vi "Counter - Count Edges Test.vi"(10 "Sample Rate":dbl=100000.0, 11 "Samples per Loop":i32=100) -> (1 "counts/bin":u32[](array[numeric]), 2 "raw Data":u32[](array[numeric]))   [LabVIEW 2022 SP3]
doc: "This example demonstrates how to continuously read back the number of digital edges that have been counted by a counter input. It uses an external clock so that the samples of the count register occur at regular intervals. If you do not need deterministic sampling of the count register, refer instead to the Count Edges example which does not use an external clock.\n\nFor instructions on how to connect your signals to the DAQ device, refer to your device documentation."
uses:
  <vilib>/Utility/error.llb/DialogType.ctl
  <vilib>/DAQmx/read.llb/DAQmx Read (Counter 1D U32 1Chan NSamp).vi
  <vilib>/DAQmx/create/channels.llb/DAQmx Create Channel (CO-Pulse Generation-Frequency).vi
  <vilib>/DAQmx/configure/timing.llb/DAQmx Timing (Implicit).vi
  <vilib>/DAQmx/create/channels.llb/DAQmx Create Channel (CI-Count Edges).vi
  <vilib>/DAQmx/configure/timing.llb/DAQmx Timing (Sample Clock).vi
  <vilib>/DAQmx/miscellaneous.llb/DAQmx Fill In Error Info.vi
  <resource>/objmgr/daqmx.rc
panel:
  out "max value":u32
  in  "Input Terminal":tag="/Dev1/PFI3"
  in  "Counter":tag="Dev1/ctr1"
  in  "Sample Clock Source":tag="/Dev1/PFI12"
  # "Channel Settings"
  # "Acquired Data"
  # "Timing Settings"
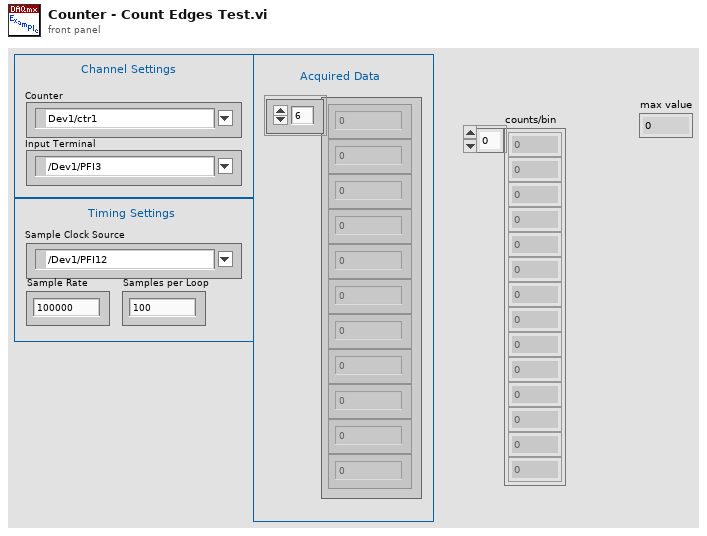
[diagram p1: front panel]
types:
  T1 = typedef "DialogType.ctl" = u16
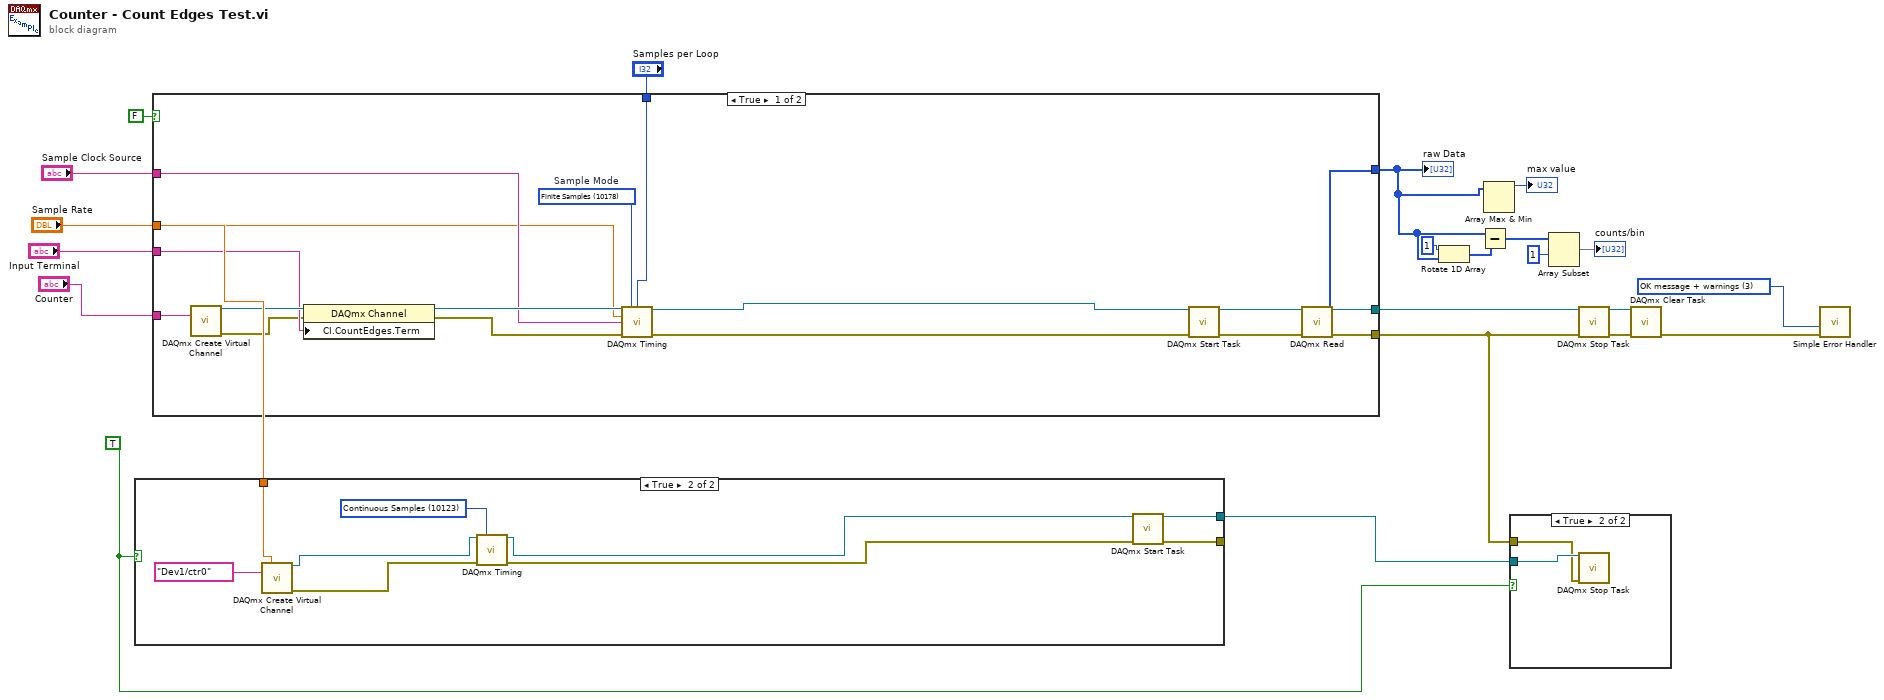
[diagram p0: block diagram]
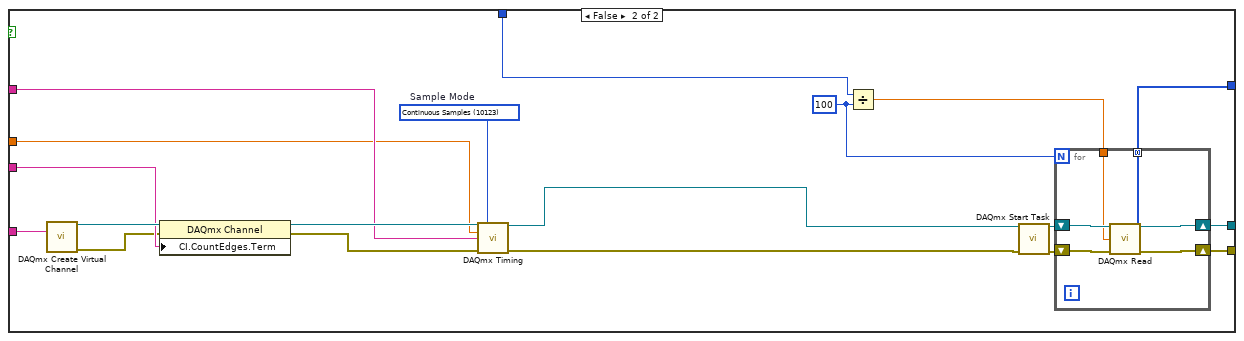
[diagram p2: hidden frame]
diagram:
  w13 = TRUE
  w16 = T1 3 items=["no dialog", "OK message", "continue or stop message", "OK message + warnings", "continue/stop + warnings"] ("type of dialog (OK msg:1)")
  n1 = case shown="True" w13 {
    tunnel: "Sample Rate" -> [_ w30]
    tunnel: [_ w28] -> w15
    tunnel: [_ w27] -> _
    frame False {
    }
    frame True {
      w24 = 10123 items=["Finite Samples"=10178, "Continuous Samples"=10123, "Hardware Timed Single Point"=12522] ("sample mode")
      n2 = call-poly <vilib>:"DAQmx Create Virtual Channel.vi"("frequency"=w30, "counter"=tag "Dev1/ctr0") -> ("task out"=w26:refnum<k21>, "error out"=w23:errorcluster)  [unwired: 12 in]
      n3 = call-poly <vilib>:"DAQmx Timing.vi"("task/channels in"=w26, "sample mode"=w24, "error in"=w23) -> ("task out"=w25:refnum<k21>, "error out"=w22:errorcluster)  [unwired: 11 in]
      n4 = call <vilib>:"DAQmx Start Task.vi"("task/channels in"=w25, "error in"=w22) -> ("task out"=w28:refnum<k21>, "error out"=w27:errorcluster)  [unwired: 12 in]
    }
  }
  n5 = case shown="True" FALSE {
    tunnel: "Counter" -> [w44 w63]
    tunnel: "Input Terminal" -> [w40 w59]
    tunnel: [w38 w57] -> w18
    tunnel: [w37 w56] -> w7
    tunnel: "Samples per Loop" -> [w36 w53]
    tunnel: [w35 w55] -> w1
    tunnel: "Sample Clock Source" -> [w34 w54]
    tunnel: "Sample Rate" -> [w31 w48]
    frame True {
      w47 = 10178 items=["Finite Samples"=10178, "Continuous Samples"=10123, "Hardware Timed Single Point"=12522]  # Sample Mode
      n6 = call-poly <vilib>:"DAQmx Create Virtual Channel.vi"("counter"=w44) -> ("task out"=w43:refnum<k21>, "error out"=w39:errorcluster)  [unwired: 13 in]
      n7 = property class="DAQmx Channel"(reference=w43, error in=w39, "CI.CountEdges.Term"=w40) -> (reference out=w42:refnum<k21>, error out=w41:errorcluster)
      n8 = call-poly <vilib>:"DAQmx Timing.vi"("task/channels in"=w42, "sample mode"=w47, "samples per channel"=w36, "rate"=w31, "source"=w34, "error in"=w41) -> ("task out"=w33:refnum<k21>, "error out"=w32:errorcluster)  [unwired: 8 in]
      n9 = call <vilib>:"DAQmx Start Task.vi"("task/channels in"=w33, "error in"=w32) -> ("task out"=w46:refnum<k21>, "error out"=w45:errorcluster)  [unwired: 12 in]
      n10 = call-poly <vilib>:"DAQmx Read.vi"("task/channels in"=w46, "error in"=w45) -> ("task out"=w38:refnum<k21>, "data"=w35:u32[], "error out"=w37:errorcluster)  [unwired: 11 in]
    }
    frame False {
      w52 = 100 ("y")
      w66 = 10123 items=["Finite Samples"=10178, "Continuous Samples"=10123, "Hardware Timed Single Point"=12522]  # Sample Mode
      n11 = call-poly <vilib>:"DAQmx Create Virtual Channel.vi"("counter"=w63) -> ("task out"=w62:refnum<k21>, "error out"=w58:errorcluster)  [unwired: 13 in]
      n12 = property class="DAQmx Channel"(reference=w62, error in=w58, "CI.CountEdges.Term"=w59) -> (reference out=w61:refnum<k21>, error out=w60:errorcluster)
      n13 = call-poly <vilib>:"DAQmx Timing.vi"("task/channels in"=w61, "sample mode"=w66, "rate"=w48, "source"=w54, "error in"=w60) -> ("task out"=w49:refnum<k21>, "error out"=w50:errorcluster)  [unwired: 9 in]
      n14 = Divide(x=w53, y=w52) -> (x/y=w51:dbl)
      n15 = call <vilib>:"DAQmx Start Task.vi"("task/channels in"=w49, "error in"=w50) -> ("task out"=w65:refnum<k21>, "error out"=w64:errorcluster)  [unwired: 12 in]
      n16 = for {
        N: w52 -> [_]
        tunnel: [w68] -> w55 mode=concatenating
        shift-right: [w70] -> w57
        shift-left: w65 -> [w72]
        shift-right: [w69] -> w56
        shift-left: w64 -> [w71]
        tunnel: w51 -> [w67]
        n17 = call-poly <vilib>:"DAQmx Read.vi"("task/channels in"=w72, "number of samples per channel"=w67, "error in"=w71) -> ("task out"=w70:refnum<k21>, "data"=w68:u32[], "error out"=w69:errorcluster)  [unwired: 10 in]
      }
    }
  }
  "raw Data" <- w1
  n18 = Rotate 1D Array(1:w1, 2:1 ("n")) -> (0:w5:u32[])
  n19 = Subtract(x=w1, y=w5) -> (x-y=w4:u32[])
  n20 = Array Max & Min(array=w1) -> (max value=→"max value":u32)  [unwired: 3 out]
  n21 = case shown="True" w13 {
    tunnel: w15 -> [_ w74]
    tunnel: w7 -> [_ w73]
    frame False {
    }
    frame True {
      n22 = call <vilib>:"DAQmx Stop Task.vi"("task/channels in"=w74, "error in"=w73) -> ()  [unwired: 12 in, 2 out]
    }
  }
  n23 = Array Subset(array=w4, index=1) -> (→"counts/bin":u32[])  [unwired: 1 in]
  n24 = call <vilib>:"DAQmx Stop Task.vi"("task/channels in"=w18, "error in"=w7) -> ("task out"=w17:refnum<k21>, "error out"=w10:errorcluster)  [unwired: 12 in]
  n25 = call <vilib>:"DAQmx Clear Task.vi"("task in"=w17, "error in"=w10) -> ("error out"=w21:errorcluster)  [unwired: 13 in]
  n26 = call <vilib>:"Simple Error Handler.vi"("type of dialog (OK msg:1)"=w16, "error in (no error)"=w21) -> ()  [unwired: 3 in, 5 out]
